vi "CanChannelOpen.vi"(3 "error in":errorcluster {"code" format="%.0x"}, 4 "Exclusive":bool, 5 "CAN Number":u32 max=31 step=1, 6 "Device Handle":u32 format="%x") -> (0 "error out":errorcluster {"code" format="%.0x"}, 2 "CAN Channel Handle":u32 format="%x")   [LabVIEW 2012]
doc: "Opens a CAN channel on the specified VCI device."
uses:
  vcilva.dll
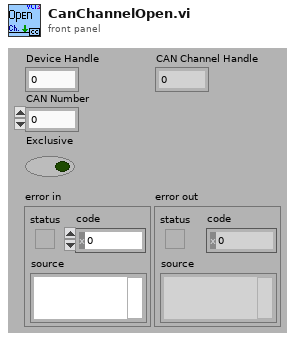
[diagram p1: front panel]
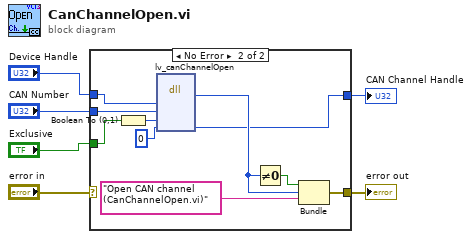
[diagram p0: block diagram]
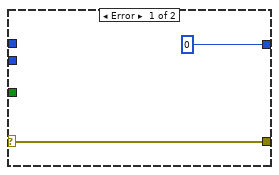
[diagram p2: hidden frame]
diagram:
  n1 = case shown="No Error" "error in" {
    selector: "error in" -> [w8 _]
    tunnel: "Device Handle" -> [_ w18]
    tunnel: "CAN Number" -> [_ w17]
    tunnel: "Exclusive" -> [_ w11]
    tunnel: [u32 0 ("hCanCtrl") w9] -> w2
    tunnel: [w8 w15] -> w1
    frame Error {
    }
    frame No Error {
      n2 = Boolean To (0,1)(Boolean=w11) -> (0, 1=w12:i16)
      n3 = dll-call lib="vcilva.dll" fn="lv_canChannelOpen"("hDevice"=w18, "dwCanNo"=w17, "fExclusive"=w12, "hCanChn"=u32 0 ("hCanChan")) -> (w13:i32, "hCanChn"=w9:u32)  [unwired: 6 in, 2 out]
      n4 = Not Equal To 0?(x=w13) -> (x != 0?=w14:bool)
      n5 = Bundle(w14, w13, "Open CAN channel (CanChannelOpen.vi)") -> (w15:errorcluster)  [unwired: 1 in]
    }
  }
  "CAN Channel Handle" <- w2
  "error out" <- w1
